vi "Create.vi"(8 "error in (no error)":errorcluster) -> (0 "error out":errorcluster, 3 "timing status pointer":refnum<class "Timing Status Pointer.lvclass">)   [LabVIEW 2021, in "DSF Core.lvlib" / "Timing Status Pointer.lvclass"]
uses:
  Timing Status Pointer.lvclass
  C:/Program Files/National Instruments/LabVIEW 2021/vi.lib/NI/Memory Manager/Classes/Pointer/Pointer.lvclass
  <vilib>/NI/Memory Manager/Classes/Pointer/Pointer.lvclass/Pointer.ctl
  <vilib>/NI/Memory Manager/Classes/Pointer/Set Address.vi
  <vilib>/NI/Memory Manager/Classes/Pointer/Set Size.vi
  <vilib>/NI/Memory Manager/Classes/Pointer/Set Internal.vi
  <vilib>/NI/Memory Manager/Classes/Pointer/Pointer.lvclass
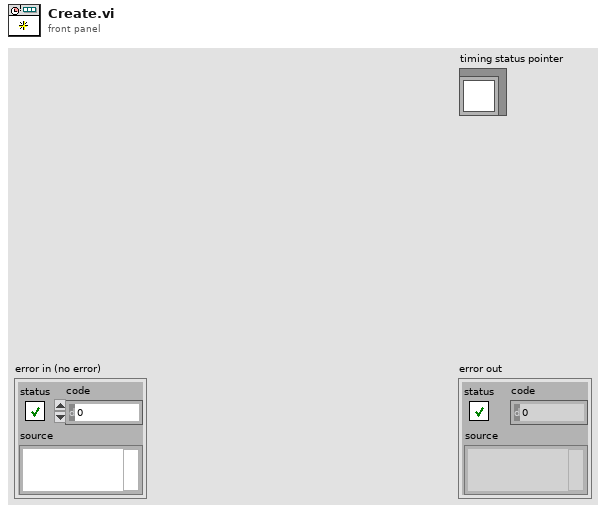
[diagram p1: front panel]
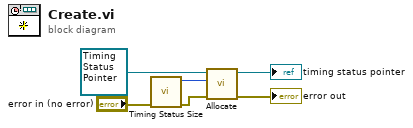
[diagram p0: block diagram]
diagram:
  n1 = call "Timing Status Size.vi"("error in (no error)"="error in (no error)") -> ("error out"=w1:errorcluster, "size"=w3:u64)  [unwired: 9 in]
  n2 = call <vilib>:"Allocate.vi"("error in (no error)"=w1, "size"=w3, "Pointer type"=refnum<class "Timing Status Pointer.lvclass"> refnum ("timing status pointer in")) -> ("error out"=→"error out":errorcluster, "Pointer out"=→"timing status pointer":refnum<class "Timing Status Pointer.lvclass">)  [unwired: 7 in]
